vi "Dust_Type_Query.vi"(8 "error in (no error)":errorcluster, 11 "Dust Name":string) -> (0 "error out":errorcluster, 3 "Dust Type Array":T1[](array[typedef]))   [LabVIEW 2013]
uses:
  Controls/Dust_list.ctl
  <vilib>/addons/database/_DB Variant To Data/Database Variant To Data.xnode
panel:
  out "Query in Standard Format":string
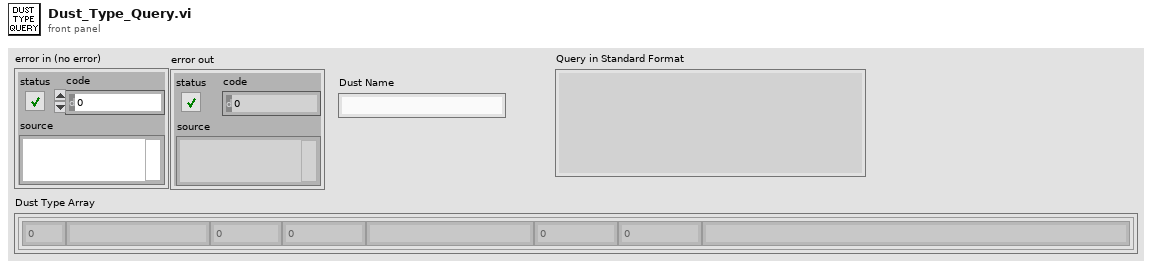
[diagram p1: front panel]
types:
  T1 = typedef "dust_list.ctl" = cluster{"id_dust_type":i32, "dust_name":string, "dust_density":dbl, "source_weight":dbl, "size":string, "bottle_weight":dbl, "dust_mass":dbl, "comments":string}
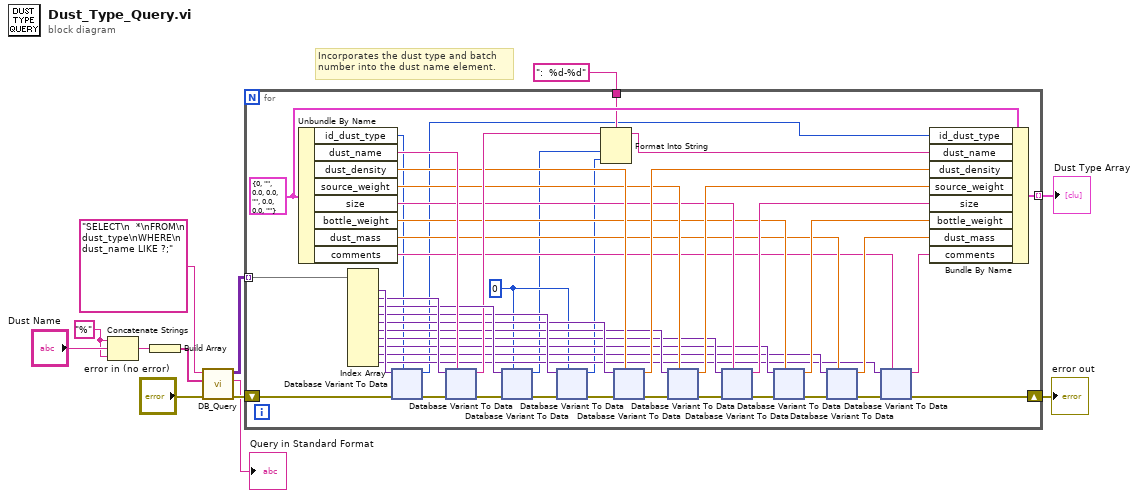
[diagram p0: block diagram]
diagram:
  w2 = "%" ("string")
  # "Incorporates the dust type and batch\nnumber into the dust name element."
  n1 = Concatenate Strings(w2, "Dust Name", w2) -> (w4:string)
  n2 = Build Array(w4) -> (w11:string[])
  n3 = call "DB_Query.vi"("error in (no error)"="error in (no error)", "Parameters"=w11, "Parameterized Query"="SELECT\n  *\nFROM\n  dust_type\nWHERE\n  dust_name LIKE ?;") -> ("error out"=w10:errorcluster, "Query in Standard Format"=→"Query in Standard Format":string, "Results"=w8:variant[][])  [unwired: 6 in]
  n4 = for {
    shift-right: [w18] -> w9
    shift-left: w10 -> [w54]
    tunnel: w8 -> [w57] mode=indexing
    tunnel: [w55] -> w7 mode=indexing
    tunnel: ":  %d-%d" -> [w46]
    w17 = 0 ("data")
    w56 = T1 {"id_dust_type"=0, "dust_name"="", "dust_density"=0.0, "source_weight"=0.0, "size"="", "bottle_weight"=0.0, "dust_mass"=0.0, "comments"=""} ("Cluster")
    n5 = Unbundle By Name(w56) -> ("id_dust_type"=w14:i32, "dust_name"=w50:string, "dust_density"=w40:dbl, "source_weight"=w37:dbl, "size"=w32:string, "bottle_weight"=w29:dbl, "dust_mass"=w24:dbl, "comments"=w20:string)
    n6 = Index Array(array=w57) -> (element #1=w53:variant, element #2=w51:variant, element #3=w48:variant, element #4=w43:variant, element #5=w41:variant, element #6=w36:variant, element #7=w33:variant, element #8=w28:variant, element #9=w25:variant, element #10=w21:variant)  [unwired: 10 in]
    n7 = xnode "Database Variant To Data"("database variant"=w53, "error in (no error)"=w54, "type"=w14) -> ("data"=w13:i32, "error out"=w52:errorcluster)
    n8 = xnode "Database Variant To Data"("database variant"=w51, "error in (no error)"=w52, "type"=w50) -> ("data"=w45:string, "error out"=w49:errorcluster)
    n9 = xnode "Database Variant To Data"("database variant"=w48, "error in (no error)"=w49, "type"=w17) -> ("data"=w16:i32, "error out"=w44:errorcluster)
    n10 = xnode "Database Variant To Data"("database variant"=w43, "error in (no error)"=w44, "type"=w17) -> ("data"=w15:i32, "error out"=w42:errorcluster)
    n11 = Format Into String(format string=w46, initial string=w45, w16, w15) -> (resulting string=w47:string)  [unwired: 1 in, 1 out]
    n12 = xnode "Database Variant To Data"("database variant"=w41, "error in (no error)"=w42, "type"=w40) -> ("data"=w39:dbl, "error out"=w38:errorcluster)
    n13 = xnode "Database Variant To Data"("database variant"=w36, "error in (no error)"=w38, "type"=w37) -> ("data"=w34:dbl, "error out"=w35:errorcluster)
    n14 = xnode "Database Variant To Data"("database variant"=w33, "error in (no error)"=w35, "type"=w32) -> ("data"=w31:string, "error out"=w30:errorcluster)
    n15 = xnode "Database Variant To Data"("database variant"=w28, "error in (no error)"=w30, "type"=w29) -> ("data"=w27:dbl, "error out"=w26:errorcluster)
    n16 = xnode "Database Variant To Data"("database variant"=w25, "error in (no error)"=w26, "type"=w24) -> ("data"=w23:dbl, "error out"=w22:errorcluster)
    n17 = xnode "Database Variant To Data"("database variant"=w21, "error in (no error)"=w22, "type"=w20) -> ("data"=w19:string, "error out"=w18:errorcluster)
    n18 = Bundle By Name(cluster=w56, "id_dust_type"=w13, "dust_name"=w47, "dust_density"=w39, "source_weight"=w34, "size"=w31, "bottle_weight"=w27, "dust_mass"=w23, "comments"=w19) -> (w55:T1)
  }
  "error out" <- w9
  "Dust Type Array" <- w7
